vi "DMD_Device_Alloc_.vi"(6 "Master/Slave Mode":i32, 7 "Inversion":i32) -> (0 "error out":errorcluster, 2 "DeviceIdPtr":u32, 3 "DLP Type":i32)   [LabVIEW 2020]
uses:
  <vilib>/Utility/error.llb/Error Cluster From Error Code.vi
  <userlib>/alp4395/alp4395.dll
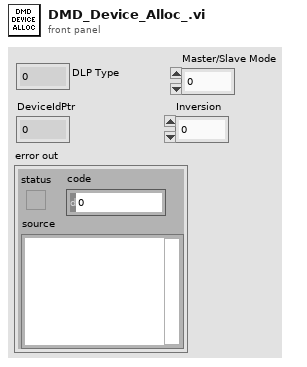
[diagram p1: front panel]
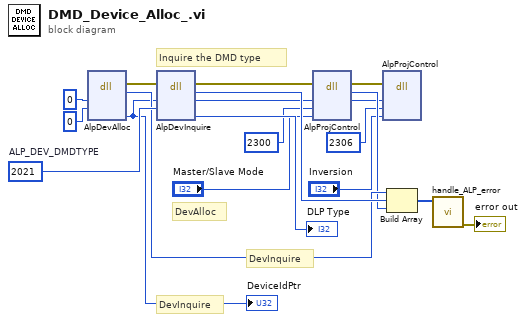
[diagram p0: block diagram]
diagram:
  w15 = 2021  # ALP_DEV_DMDTYPE
  # "DevInquire"
  # "Inquire the DMD type"
  # "DevInquire"
  # "DevAlloc"
  n1 = dll-call lib="C:/Program Files (x86)/National Instruments/LabVIEW 2020/user.lib/alp4395/alp4395.dll" fn="AlpDevAlloc"("DeviceNum"=0, "InitFlag"=0) -> (error out=w12:errorcluster, "return type"=w11:i32, "DeviceIdPtr"=w10:u32)  [unwired: 6 in, 1 out]
  "DeviceIdPtr" <- w10
  n2 = dll-call lib="C:/Program Files (x86)/National Instruments/LabVIEW 2020/user.lib/alp4395/alp4395.dll" fn="AlpDevInquire"(error in=w12, "DeviceId"=w10, "InquireType"=w15) -> (error out=w9:errorcluster, "return type"=w18:i32, "DeviceId"=w8:u32, "UserVar"=→"DLP Type":i32)  [unwired: 4 in, 1 out]
  n3 = dll-call lib="C:/Program Files (x86)/National Instruments/LabVIEW 2020/user.lib/alp4395/alp4395.dll" fn="AlpProjControl" ("alpD40.dll:AlpDevInquire")(error in=w9, "DeviceId"=w8, "ControlType"=2300, "ControlVaule"="Master/Slave Mode") -> (error out=w4:errorcluster, "return type"=w5:i32, "DeviceId"=w3:u32)  [unwired: 4 in, 1 out]
  n4 = dll-call lib="C:/Program Files (x86)/National Instruments/LabVIEW 2020/user.lib/alp4395/alp4395.dll" fn="AlpProjControl" ("alpD40.dll:AlpDevInquire")(error in=w4, "DeviceId"=w3, "ControlType"=2306, "ControlVaule"="Inversion") -> ()  [unwired: 6 in, 2 out]
  n5 = Build Array(w11, w18, w5) -> (w17:i32[])
  n6 = call "handle_ALP_error.vi"("Return Codes"=w17) -> ("error out"=→"error out":errorcluster)  [unwired: 10 in]
